vi "LIDAR_FindBall.vi"(10 "Front/Back":T1, 11 "Data Highway Out 2":T2={"New Image"=refnum, "Session Out"="", "LIDAR VISA Name"="", "Phidget Device Out"=0, "Lidar Data"=[], "polar attributes"={"maximum"=0.0, "minimum"=0.0, "clip to min"=FALSE, "log?(F)"=FALSE, "grid color"=6710886, "plot color"=65280, "fmt and prec"={"format"=enum."Decimal", "precision"=0}, "visible section"=8}, "Debug Statement"="", "Servo Angles"={"Angle X"=0.0, "Angle Y"=0.0}, "ColorPlane"=refnum, "Threshold"=refnum, "PartFilt"=refnum, "Processed Image"=refnum, "Magnitude"=[], "Direction"=[]} {"polar attributes"."minimum" format="%0.2f"; "polar attributes"."maximum" format="%0.2f"}) -> (2 "Ball Locations":dbl[](array[numeric]))   [LabVIEW 2014]
uses:
  controls/Data.ctl
  <vilib>/vision/Image Controls.llb/IMAQ Image.ctl
  <vilib>/userdefined/High Color/IMAQdx.ctl
  controls/FrontBack.ctl
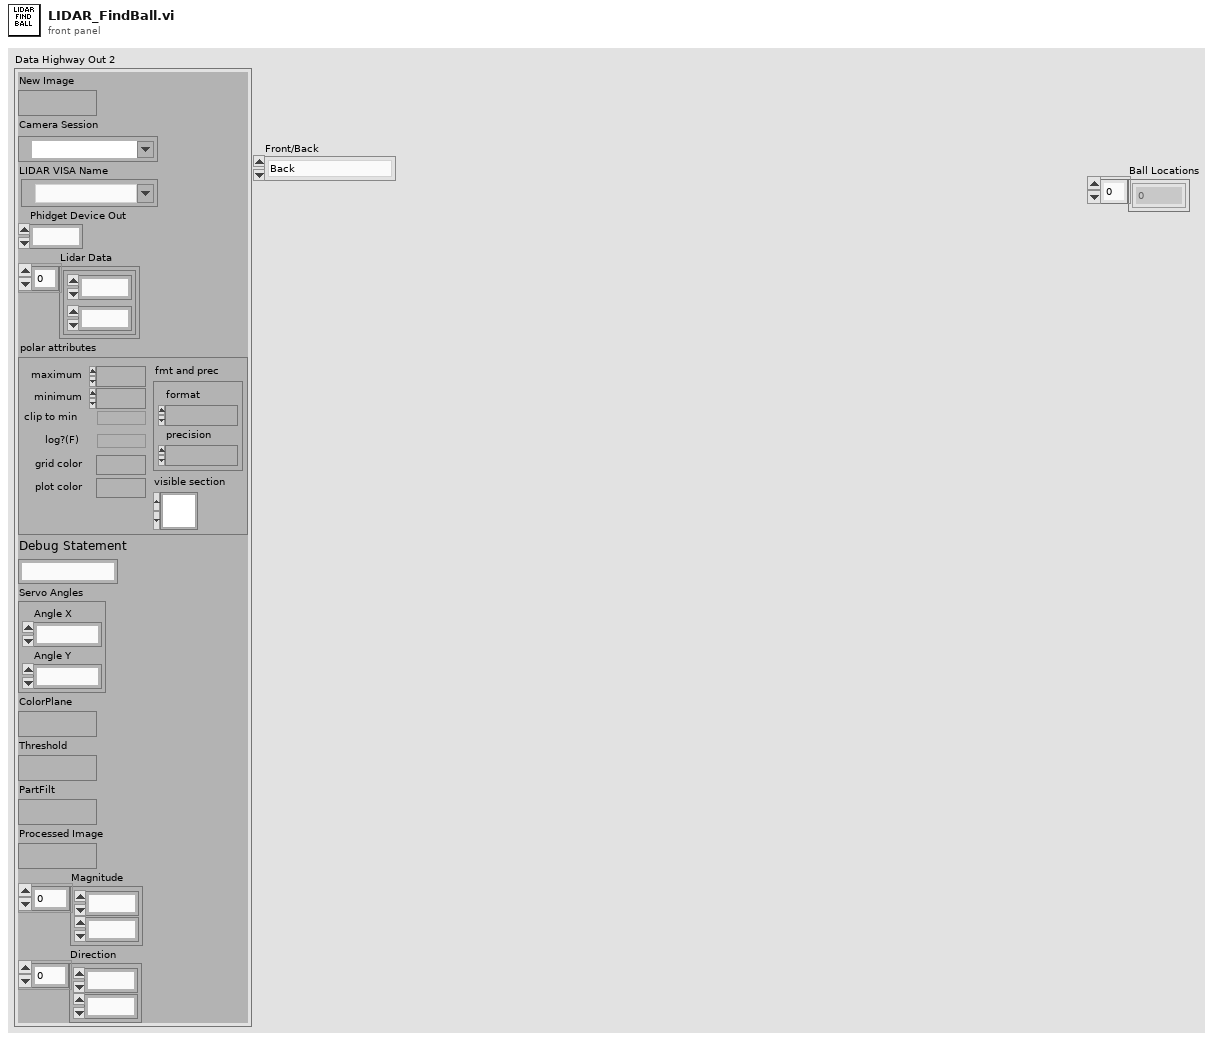
[diagram p1: front panel]
types:
  T1 = typedef "FrontBack.ctl" = enum16{"Back", "Front"}
  T2 = typedef "Data.ctl" = cluster{"New Image":T3, "Session Out":T4, "LIDAR VISA Name":refnum<visa-resource-name>, "Phidget Device Out":i32, "Lidar Data":cluster{dbl, dbl}[], "polar attributes":cluster{"maximum":dbl, "minimum":dbl, "clip to min":bool, "log?(F)":bool, "grid color":u32, "plot color":u32, "fmt and prec":cluster{"format":enum8{"Decimal", "Scientific", "Engineering", "Binary", "Octal", "Hex"}, "precision":u8}, "visible section":u16}, "Debug Statement":string, "Servo Angles":cluster{"Angle X":dbl, "Angle Y":dbl}, "ColorPlane":T3, "Threshold":T3, "PartFilt":T3, "Processed Image":T3, "Magnitude":dbl[], "Direction":dbl[]}
  T3 = typedef "IMAQ Image.ctl" = refnum<image>
  T4 = typedef "IMAQdx.ctl" = refnum<k21>
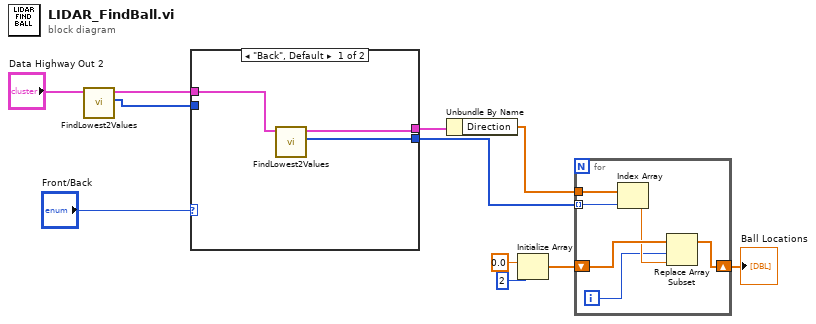
[diagram p0: block diagram]
diagram:
  n1 = call "FindLowest2Values.vi"("Data Highway Out 2"="Data Highway Out 2") -> ("Index of vals"=w8:i64[], "Data Highway Out 3"=w9:T2)  [unwired: 9 in]
  n2 = case shown="\"Back\", Default" "Front/Back" {
    tunnel: w9 -> [w14 w15]
    tunnel: w8 -> [_ w16]
    tunnel: [w13 w16] -> w7
    tunnel: [w12 w15] -> w2
    frame "Back", Default {
      n3 = call "FindLowest2Values.vi"("Data Highway Out 2"=w14) -> ("Index of vals"=w13:i64[], "Data Highway Out 3"=w12:T2)  [unwired: 9 in]
    }
    frame "Front" {
    }
  }
  n4 = Unbundle By Name(w2) -> ("Direction"=w6:dbl[])
  n5 = Initialize Array(0.0 ("element"), 2 ("dimension size")) -> (w3:dbl[])
  n6 = for {
    tunnel: w7 -> [w22] mode=indexing
    tunnel: w6 -> [w21]
    shift-right: [w18] -> w1
    shift-left: w3 -> [w20]
    i -> [w17]
    n7 = Index Array(array=w21, index=w22) -> (element=w19:dbl)
    n8 = Replace Array Subset(array=w20, new element=w19, index=w17) -> (w18:dbl[])
  }
  "Ball Locations" <- w1
